vi "4_PM.vi"() -> ()   [LabVIEW 2026]
uses:
  <vilib>/measure/maresamp.llb/Align M + N Waveforms (single shot).vi
  <vilib>/measure/NI_MAPro.lvlib
panel:
  out "PM Result":waveform(dbl)[](graph) caption="cos carrier"
  out "message":dynamicdata(graph) caption="message\nmessage"
  out "cos carrier":dynamicdata(graph)
  in  "y":dbl
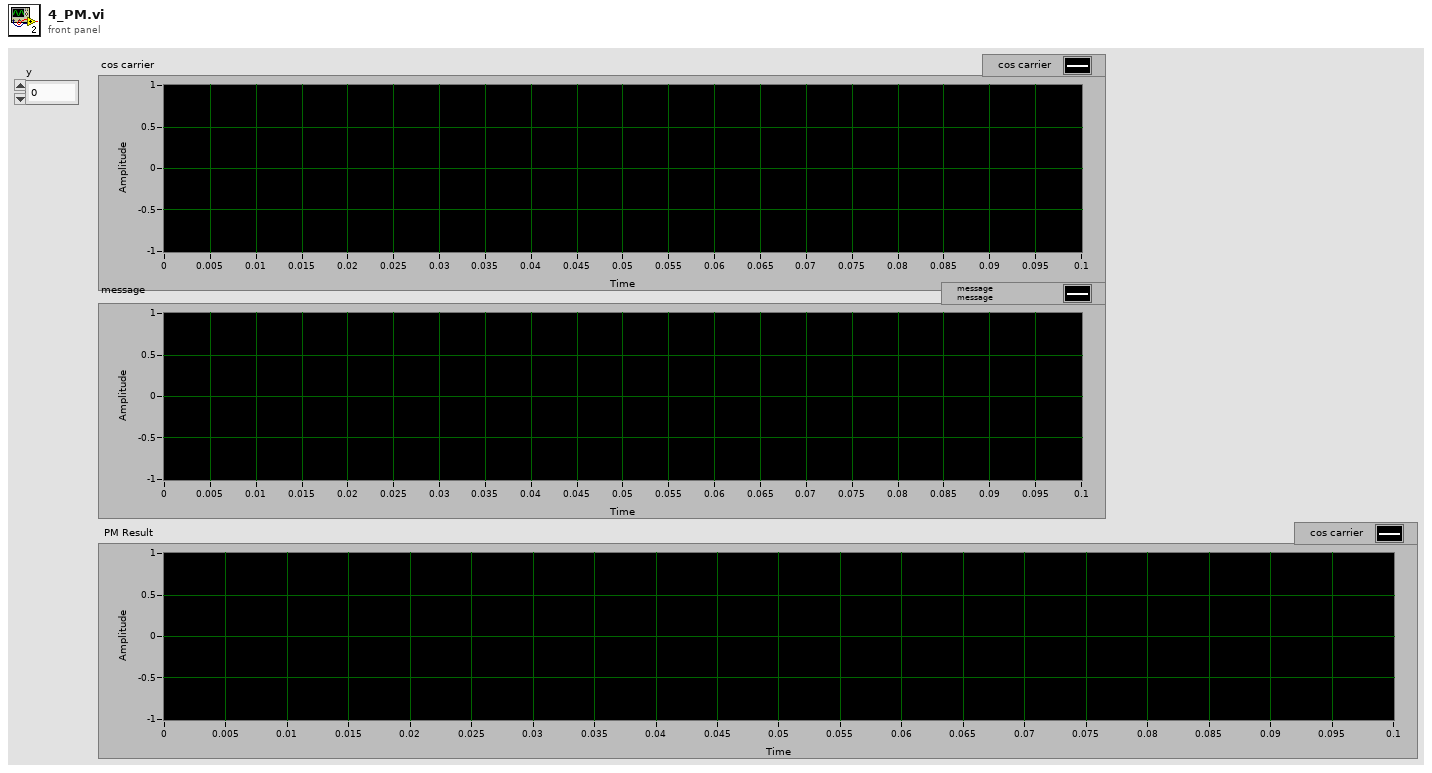
[diagram p1: front panel]
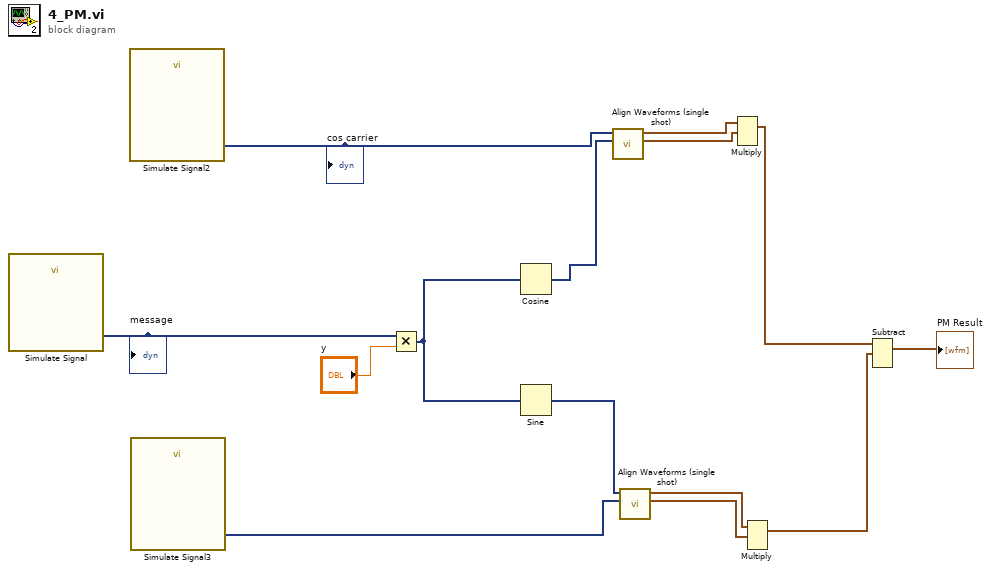
[diagram p0: block diagram]
diagram:
  n1 = call "Simulate Signal"() -> ("message\nmessage"=w14:dynamicdata)  [unwired: 14 in, 1 out]
  "message" <- w14
  n2 = call "Simulate Signal2"() -> ("cos carrier"=w11:dynamicdata)  [unwired: 14 in, 1 out]
  "cos carrier" <- w11
  n3 = call "Simulate Signal3"() -> ("sin carrier"=w9:dynamicdata)  [unwired: 14 in, 1 out]
  n4 = Multiply(x=w14, y="y") -> (x*y=w12:dynamicdata)
  n5 = Cosine(x=w12) -> (cos(x)=w10:dynamicdata)
  n6 = Sine(x=w12) -> (sin(x)=w8:dynamicdata)
  n7 = call-poly <vilib>:"Align Waveforms (single shot).vi"("N waveforms in"=w10, "M waveforms in"=w11) -> ("N aligned waveforms out"=w7:waveform(dbl)[], "M aligned waveforms out"=w6:waveform(dbl)[])  [unwired: 7 in, 1 out]
  n8 = call-poly <vilib>:"Align Waveforms (single shot).vi"("N waveforms in"=w9, "M waveforms in"=w8) -> ("N aligned waveforms out"=w5:waveform(dbl)[], "M aligned waveforms out"=w4:waveform(dbl)[])  [unwired: 7 in, 1 out]
  n9 = Multiply(1:w7, 2:w6) -> (0:w3:waveform(dbl)[])  [unwired: 1 in, 1 out]
  n10 = Multiply(1:w5, 2:w4) -> (0:w2:waveform(dbl)[])  [unwired: 1 in, 1 out]
  n11 = Subtract(1:w2, 2:w3) -> (0:→"PM Result":waveform(dbl)[])  [unwired: 1 in, 1 out]
